vi "t2.vi"() -> ()   [LabVIEW 2024]
panel:
  out "Q12-T2":cluster{dbl[], dbl[]}(graph)
  out "Q2-T2":cluster{dbl[], dbl[]}(graph)
  out "Q1-T1":cluster{dbl[], dbl[]}(graph)
  out "2D Picture 2":picture
  in  "L 2":dbl(slide)=80.0 scale=0.0..200.0
  in  "L 1":dbl(slide)=80.0 scale=0.0..200.0
  in  "file (use dialog)":path
  out "end effector":cluster{dbl, dbl}={159.01647214211073, 1.9100783062530127} {"?" format="%.1f"; "?" format="%#.1f"}
  out "2D Picture":picture
  in  "2D Pict origin":cluster{"x":dbl, "y":dbl}={"x"=200.0, "y"=200.0}
  # "mm"
  # "mm"
  # "mm"
  # "mm"
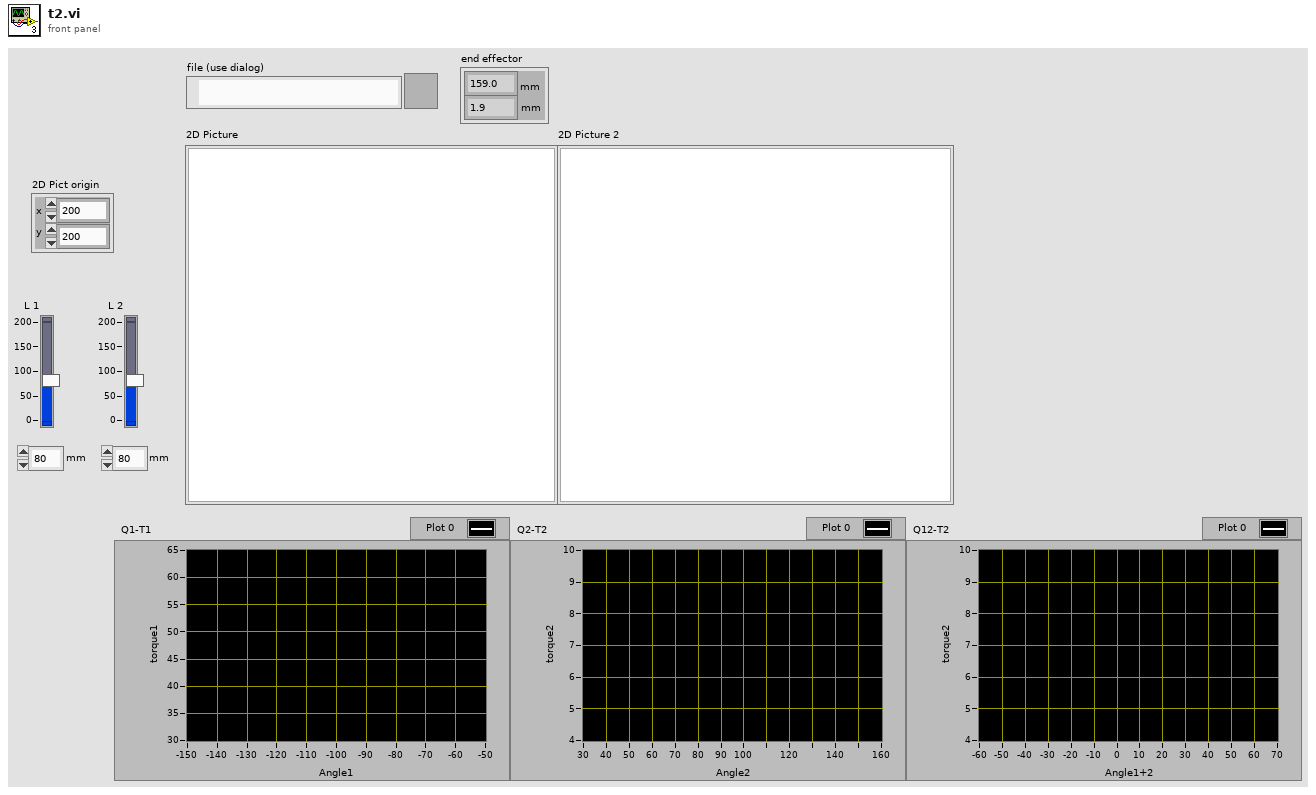
[diagram p1: front panel]
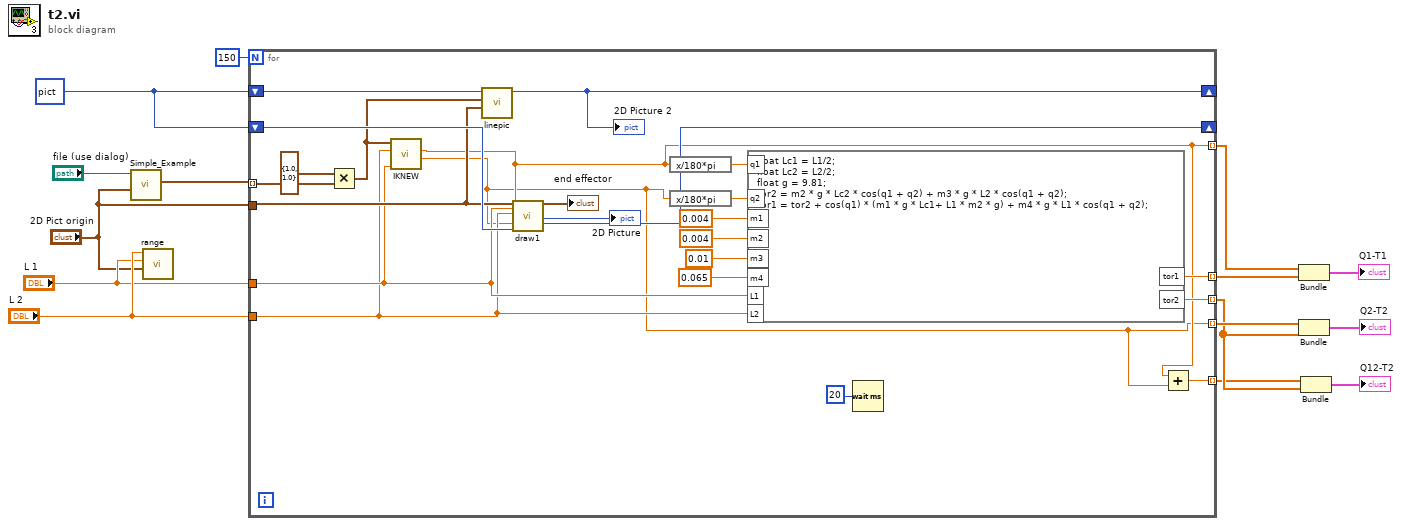
[diagram p0: block diagram]
diagram:
  w10 = picture data[5B] ("new picture")
  n1 = call <userlib>:"Simple_Example.vi"("2D Pict origin"="2D Pict origin", "file (use dialog)"="file (use dialog)") -> ("xy coord"=w15:cluster{"x":dbl, "y":dbl}[])  [unwired: 8 in, 1 out]
  n2 = call "range.vi"("2D Pict origin"="2D Pict origin", "L 1"="L 1", "L 2"="L 2") -> ()  [unwired: 8 in, 1 out]
  n3 = for {
    N: 150 -> [_]
    tunnel: w15 -> [w32] mode=indexing
    tunnel: "2D Pict origin" -> [w30]
    shift-right: [w34] -> _
    shift-left: w10 -> [w36]
    shift-right: [w29] -> _
    shift-left: w10 -> [w38]
    tunnel: "L 1" -> [w25]
    tunnel: "L 2" -> [w24]
    tunnel: [w23] -> w5 mode=indexing
    tunnel: [w22] -> w2 mode=indexing
    tunnel: [w18] -> w6 mode=indexing
    tunnel: [w17] -> w4 mode=indexing
    tunnel: [w16] -> w1 mode=indexing
    n4 = Multiply(x=cluster{dbl, dbl} {1.0, 1.0}, y=w32) -> (x*y=w31:cluster{dbl, dbl})
    n5 = call "IKNEW.vi"("L1"=w25, "L2"=w24, "coordinates"=w31) -> ("theta21"=w17:dbl, "theta11"=w18:dbl)  [unwired: 7 in]
    n6 = call "linepic.vi"("origin"=w30, "Coordinates"=w31, "shift pic"=w38) -> ("2D Picture 2"=w29:picture)  [unwired: 8 in]
    "2D Picture 2" <- w29
    n7 = call "draw1.vi"("new position"=w30, "L 1"=w25, "L 2"=w24, "Angle1"=w18, "Angle 2"=w17, "input pic in loop"=w36) -> ("end effector"=→"end effector":cluster{dbl, dbl}, "2D Picture"=→"2D Picture":picture, "shift pic"=w34:picture)  [unwired: 9 in, 2 out]
    n8 = expression code="x/180*pi"(w18) -> (w21:dbl)
    n9 = expression code="x/180*pi"(w17) -> (w20:dbl)
    n10 = formula code="float Lc1 = L1/2;\nfloat Lc2 = L2/2;\nfloat g = 9.81;\ntor2 = m2 * g * Lc2 * cos(q1 + q2) + m3 * g * L2 * cos(q1 + q2);\ntor1 = tor2 + cos(q1) * (m1 * g * Lc1+ L1 * m2 * g) + m4 * g * L1 * cos(q1 + q2);"("q1"=w21, "q2"=w20, "m1"=0.004 ("input variable"), "m2"=0.004 ("input variable"), "L1"=w25, "L2"=w24, "m3"=0.01 ("input variable"), "m4"=0.065 ("input variable")) -> ("tor1"=w23:dbl, "tor2"=w22:dbl)
    n11 = Wait (ms)(milliseconds to wait=u32 20) -> ()  [unwired: 1 out]
    n12 = Add(x=w18, y=w17) -> (x+y=w16:dbl)
  }
  n13 = Bundle(w6, w5) -> (→"Q1-T1":cluster{dbl[], dbl[]})  [unwired: 1 in]
  n14 = Bundle(w4, w2) -> (→"Q2-T2":cluster{dbl[], dbl[]})  [unwired: 1 in]
  n15 = Bundle(w1, w2) -> (→"Q12-T2":cluster{dbl[], dbl[]})  [unwired: 1 in]
